vi "Test5.vi"() -> ()   [LabVIEW 2010]
uses:
  <vilib>/MDSplus/Library/MDSplus.lvlib
panel:
  out "Float out 2":sgl
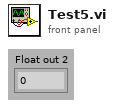
[diagram p1: front panel]
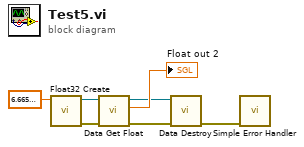
[diagram p0: block diagram]
diagram:
  n1 = call <vilib>:"Float32 Create.vi"("SGL in"=sgl 6.666 ("Value")) -> ("error out"=w5:errorcluster, "Float32 DVR out"=w6:refnum<data-value>)  [unwired: 9 in]
  n2 = call <vilib>:"Data Get Float.vi"("error in (no error)"=w5, "Data DVR in"=w6) -> ("error out"=w2:errorcluster, "SGL out"=→"Float out 2":sgl, "Data DVR out"=w3:refnum<data-value>)  [unwired: 7 in]
  n3 = call <vilib>:"Data Destroy.vi"("error in (no error)"=w2, "Data DVR in"=w3) -> ("error out"=w1:errorcluster)  [unwired: 9 in]
  n4 = call <vilib>:"Simple Error Handler.vi"("error in (no error)"=w1) -> ()  [unwired: 4 in, 5 out]
